vi "Get All Possible Shortcuts.vi"() -> (0 "All Possible Shortcuts":string[](array[string]))   [LabVIEW 2021, in "Seq Edit Quick Drop.lvlib"]
uses:
  Seq Edit Quick Drop.lvlib
  Scan Codes Mapping.vi
  <vilib>/Utility/error.llb/Trim Whitespace.vi
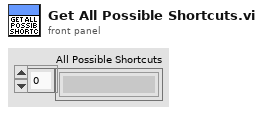
[diagram p1: front panel]
types:
  T1 = typedef "Seq Edit Quick Drop.lvlib/Key Code.ctl" = cluster{"Key":string, "Scan Code":i16}
  T2 = typedef "Seq Edit Quick Drop.lvlib/Modifiers.ctl" = enum16{"SHIFT", "CTRL", "ALT"}
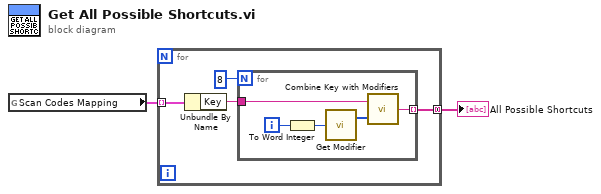
[diagram p0: block diagram]
diagram:
  n1 = global read "Scan Codes Mapping.vi" "Scan Codes Mapping"() -> (w2:T1[])
  n2 = for {
    tunnel: w2 -> [w6] mode=indexing
    tunnel: [w3] -> w1 mode=concatenating
    n3 = Unbundle By Name(w6) -> ("Key"=w4:string)
    n4 = for {
      N: 8 -> [_]
      tunnel: w4 -> [w9]
      tunnel: [w8] -> w3 mode=indexing
      i -> [w11]
      n5 = To Word Integer(number=w11) -> (16bit integer=w7:i16)
      n6 = call "Get Modifier.vi"("Modifier Code"=w7) -> ("Modifiers"=w10:T2[])  [unwired: 1 out]
      n7 = call "Combine Key with Modifiers.vi"("Modifiers"=w10, "Key"=w9) -> ("Combined"=w8:string)
    }
  }
  "All Possible Shortcuts" <- w1
